vi "Multi-line String to Array.vi"(1 "string":string) -> (0 "lines":string[](array[string]))   [LabVIEW 2020, in "openg_string.lvlib"]
doc: "Converts a multiline input <B>string</B> to a 1D array of <B>lines</B> (without EOLs). If the input string ends in an EOL, then the last line will be removed (since it is empty) -- this behavior is useful for instrument communication where the last line ends with a EOL character that we do not wish to treat as a seperate line (since it contains no data)."
uses:
  Convert EOLs/Convert EOLs (String).vi
  openg_string.lvlib
panel:
  # "[OpenG VI Tags] ***Do Not Remove***"
  # "Multi-line String to Array.vi\n\nConverts a multiline string to a 1D array of lines without EOLs.\n\nPlease visit http://www.OpenG.org to learn about the\nOpen Source LabVIEW software movement.\n\nNOTICE -- YOU MUST LEAVE THIS NOTICE IN PLACE.  PER THE TERMS OF THE LICENSE BELOW, YOU MAY SUBLICENSE THIS SOFTWARE \nIN ANY WAY THAT DOES NOT CONFLICT WITH THIS LICENSE.\n\n### BSD License (http://www.opensource.org/licenses/bsd-license.php) Begin ###\n \nCopyright (c) 2002-2007, Jim Kring <jim@jimkring.com>\n\nAll rights reserved.\n\nRedistribution and use in source and binary forms, with or without modification, are permitted provided that the following conditions are met:\n\n    * Redistributions of source code must retain the above copyright notice, this list of conditions and the following disclaimer.\n    * Redistributions in binary form must reproduce the above copyright notice, this list of conditions and the following disclaimer in the \n       documentation and/or other materials provided with the distribution.\n    * Neither the name of SciWare, James Kring, Inc., nor the names of its contributors may be used to endorse or promote products derived \n       from this software without specific prior written permission.\n\nTHIS SOFTWARE IS PROVIDED BY THE COPYRIGHT HOLDERS AND CONTRIBUTORS \"AS IS\" AND ANY EXPRESS OR IMPLIED WARRANTIES, \nINCLUDING, BUT NOT LIMITED TO, THE IMPLIED WARRANTIES OF MERCHANTABILITY AND FITNESS FOR A PARTICULAR PURPOSE ARE \nDISCLAIMED. IN NO EVENT SHALL THE COPYRIGHT OWNER OR CONTRIBUTORS BE LIABLE FOR ANY DIRECT, INDIRECT, INCIDENTAL,\n SPECIAL, EXEMPLARY, OR CONSEQUENTIAL DAMAGES (INCLUDING, BUT NOT LIMITED TO, PROCUREMENT OF SUBSTITUTE GOODS OR \nSERVICES; LOSS OF USE, DATA, OR PROFITS; OR BUSINESS INTERRUPTION) HOWEVER CAUSED AND ON ANY THEORY OF LIABILITY, \nWHETHER IN CONTRACT, STRICT LIABILITY, OR TORT (INCLUDING NEGLIGENCE OR OTHERWISE) ARISING IN ANY WAY OUT OF THE USE \nOF THIS SOFTWARE, EVEN IF ADVISED OF THE POSSIBILITY OF SUCH DAMAGE.\n\n### BSD License End ###"
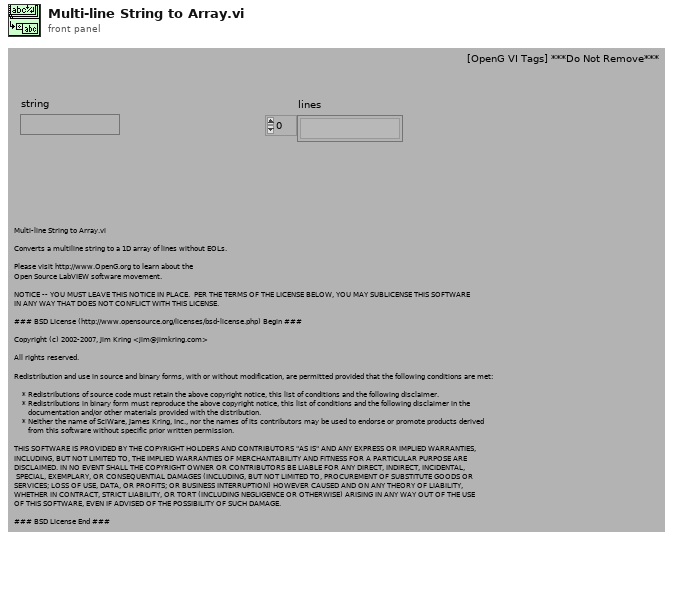
[diagram p1: front panel]
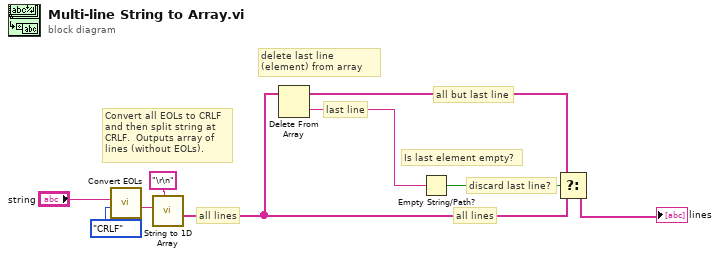
[diagram p0: block diagram]
diagram:
  # "all lines"
  # "discard last line?"
  # "delete last line (element) from array"
  # "last line"
  # "all but last line"
  # "Is last element empty?"
  # "Convert all EOLs to CRLF and then split string at CRLF.  Outputs array of lines (without EOLs)."
  # "all lines"
  n1 = call-poly "Convert EOLs.vi"("Convert to:"=enum16{"CR", "LF", "CRLF"}."CRLF", "String in"="string") -> ("String out"=w7:string)  [unwired: 9 in]
  n2 = call "String to 1D Array.vi"("delimiter (Tab)"="\r\n", "string"=w7) -> ("Array of Strings"=w6:string[])  [unwired: 9 in]
  n3 = Delete From Array(array=w6) -> (deleted portion=w3:string, array with subset deleted=w2:string[])  [unwired: 2 in]
  n4 = Empty String/Path?(string/path=w3) -> (empty?=w1:bool)
  n5 = Select(t=w2, s=w1, f=w6) -> (s? t:f=→"lines":string[])
